vi "Parse Header.vi"(8 "error in (no error)":errorcluster, 11 "Header":string[](array[string])) -> (0 "error out":errorcluster, 2 "Header String":string, 3 "Location":string)   [LabVIEW 2018, in "Receipt Parsing.lvlib"]
uses:
  Receipt Parsing.lvlib
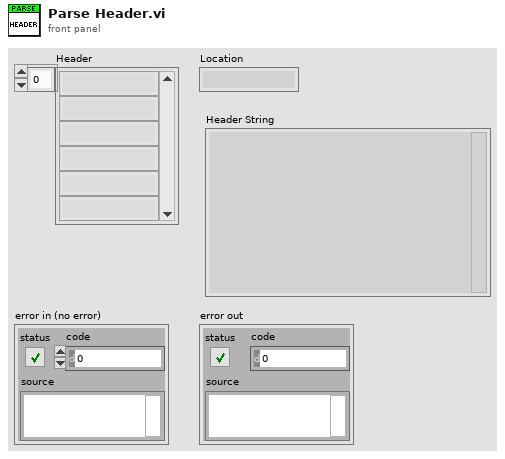
[diagram p1: front panel]
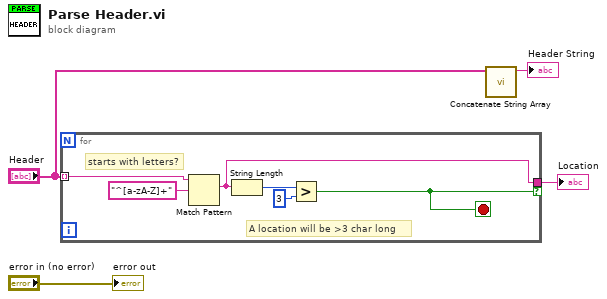
[diagram p0: block diagram]
diagram:
  n1 = for {
    tunnel: "Header" -> [w7] mode=indexing
    tunnel: [w5] -> w4 if=w6
    stop <- w6 stop-if-true
    # "A location will be >3 char long"
    # "starts with letters?"
    n2 = Match Pattern(string=w7, regular expression="^[a-zA-Z]+") -> (match substring=w5:string)  [unwired: 1 in, 3 out]
    n3 = String Length(string=w5) -> (length=w9:i32)
    n4 = Greater?(x=w9, y=3) -> (0:w6:bool)
  }
  "Location" <- w4
  n5 = call "Concatenate String Array.vi"("Array"="Header") -> ("Concatenated String"=→"Header String":string)  [unwired: 10 in]
  "error out" <- "error in (no error)"
